vi "Run Lifter.vi"(11 "MechanismMetrics in":T2) -> (3 "MechanismMetrics out":T2)   [LabVIEW 2014]
uses:
  MechanismMetrics.ctl
  Lifter States.ctl
  Auto Lifter States.ctl
  encoderData.vi
  Max and min lift velocity.vi
panel:
  in  "PID Settings":T1={"iMax"=50000.0, "iMin"=0.0, "iGain"=4e-06, "pGain"=0.0005, "dGain"=0.0, "MaxOutput"=1.0, "MinOutput"=-0.3, "AutoReset"=FALSE, "Tolerance"=100.0, "dSmoothing"=0.0}
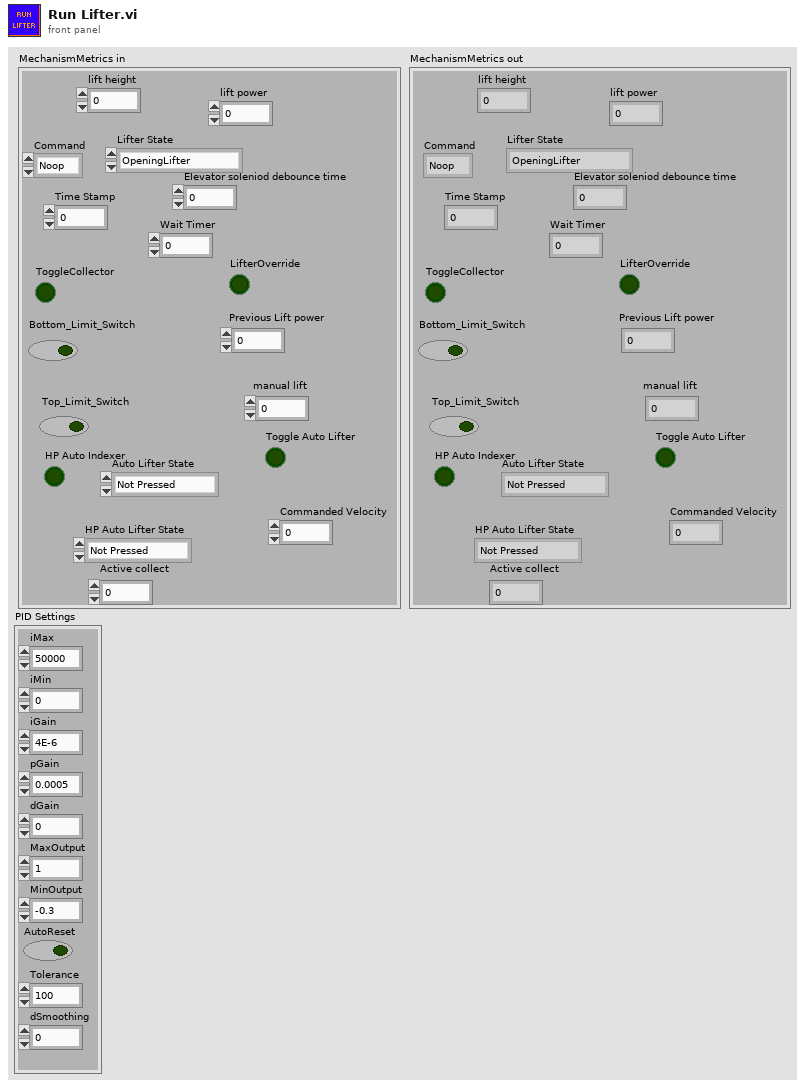
[diagram p1: front panel]
types:
  T1 = cluster{"iMax":dbl, "iMin":dbl, "iGain":dbl, "pGain":dbl, "dGain":dbl, "MaxOutput":dbl, "MinOutput":dbl, "AutoReset":bool, "Tolerance":dbl, "dSmoothing":dbl}
  T2 = typedef "MechanismMetrics.ctl" = cluster{"lift height":dbl, "Command":enum16{"Noop", "Flagged"}, "Time Stamp":u32, "ToggleCollector":bool, "Bottom_Limit_Switch ":bool, "Top_Limit_Switch":bool, "lift power":dbl, "Elevator soleniod debounce time   ":dbl, "LifterOverride":bool, "Previous Lift power":dbl, "manual lift":dbl, "Lifter State":T3, "Auto Lifter State":T4, "Toggle Auto Lifter":bool, "Wait Timer":dbl, "HP Auto Indexer":bool, "HP Auto Lifter State":T4, "Commanded Velocity":dbl, "\nActive collect":dbl}
  T3 = typedef "Lifter States.ctl" = enum16{"OpeningLifter", "LifterOpen", "ClosingLifter", "LifterClosed"}
  T4 = typedef "Auto Lifter States.ctl" = enum16{"Not Pressed", "THE_END", "WAIT_FOR_RELEASE", "Press Detected", "To Release Stacked1", "To Collect", "Open Lifter", "WAIT", "Close", "To Stack1"}
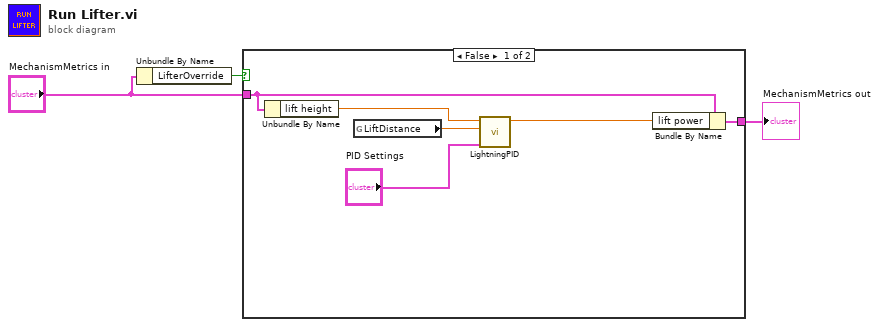
[diagram p0: block diagram]
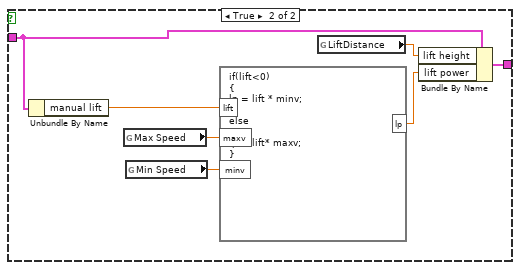
[diagram p2: hidden frame]
diagram:
  n1 = Unbundle By Name("MechanismMetrics in") -> ("LifterOverride"=w1:bool)
  n2 = case shown="False" w1 {
    tunnel: "MechanismMetrics in" -> [w6 w15]
    tunnel: [w5 w16] -> w3
    frame False {
      n3 = Unbundle By Name(w6) -> ("lift height"=w9:dbl)
      n4 = global read "encoderData.vi" "LiftDistance"() -> (w8:dbl)
      n5 = call "LightningPID.vi"("PID Settings"="PID Settings", "Position"=w8, "Set Point"=w9) -> ("Output"=w4:dbl)  [unwired: 8 in]
      n6 = Bundle By Name(cluster=w6, "lift power"=w4) -> (w5:T2)
    }
    frame True {
      n7 = Unbundle By Name(w15) -> ("manual lift"=w13:dbl)
      n8 = global read "Max and min lift velocity.vi" "Max Speed"() -> (w11:dbl)
      n9 = global read "Max and min lift velocity.vi" "Min Speed"() -> (w10:dbl)
      n10 = formula code="if(lift<0)\n{\nlp = lift * minv;\n}\nelse\n{\nlp = lift* maxv;\n}"("lift"=w13, "maxv"=w11, "minv"=w10) -> ("lp"=w12:dbl)
      n11 = global read "encoderData.vi" "LiftDistance"() -> (w14:dbl)
      n12 = Bundle By Name(cluster=w15, "lift height"=w14, "lift power"=w12) -> (w16:T2)
    }
  }
  "MechanismMetrics out" <- w3
